vi "Format Drive Letter For Net Use.vi"(10 "Drive Letter":string) -> (2 "String":string)   [LabVIEW 2017, in "G3_Build Process File Utilities.lvlib"]
uses:
  G3_Build Process File Utilities.lvlib
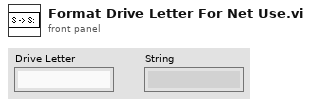
[diagram p1: front panel]
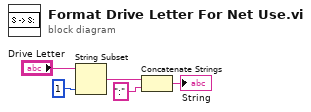
[diagram p0: block diagram]
diagram:
  n1 = String Subset(string="Drive Letter", length (rest)=1 ("length (rest)")) -> (substring=w3:string)  [unwired: 1 in]
  n2 = Concatenate Strings(w3, ":" ("string")) -> (→"String":string)
